vi "BoolToU32.vi"(11 "Boolean":bool=TRUE) -> (3 "Numeric":u32)   [LabVIEW 2012]
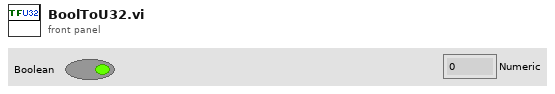
[diagram p1: front panel]
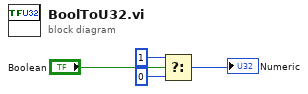
[diagram p0: block diagram]
diagram:
  n1 = Select(t=u32 1, s="Boolean", f=u32 0) -> (s? t:f=→"Numeric":u32)
